vi "Create Transfer Channels.vi"(7 "direction":T1, 8 "error in (no error)":errorcluster, 9 "Transfer ID":string, 10 "Refnum in":T3, 11 "Section Ptr":T2 format="%.0x") -> (0 "error out":errorcluster)   [LabVIEW 2017, in "Data Sharing Framework System Explorer.lvlib"]
uses:
  Data Sharing Framework System Explorer.lvlib
  dsf core/Source/DSF Configuration API/1.0.0/Public/Controls/DSF Config Data RefNum.ctl
  <vilib>/NI Veristand/Custom Device API/Custom Device Item Ref.ctl
  dsf core/Source/DSF Configuration API/1.0.0/Public/Controls/DSF Direction.ctl
  <vilib>/NI Veristand/Custom Device API/Custom Device Channel Type.ctl
  <vilib>/NI Veristand/Custom Device API/Custom Device Channel.ctl
  dsf core/Source/DSF Configuration API/1.0.0/Public/Read Item Child IDs/Read Transfer Channel IDs.vi
  <vilib>/NI Veristand/Custom Device API/Custom Device API.lvlib
  dsf core/Source/DSF Configuration API/1.0.0/DSF Configuration API.lvlib
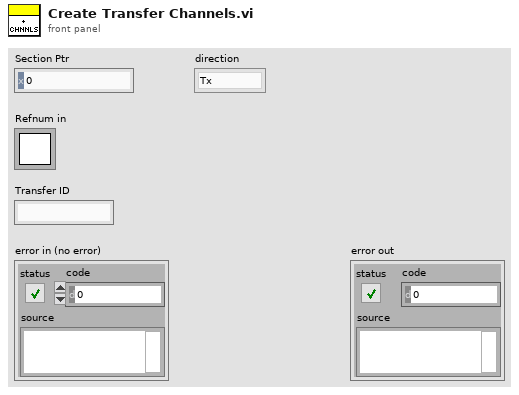
[diagram p1: front panel]
types:
  T1 = typedef "DSF Configuration API.lvlib/DSF Direction.ctl" = enum8{"Tx", "Rx"}
  T2 = typedef "Custom Device API.lvlib/Custom Device Item Ref.ctl" = u64
  T3 = typedef "DSF Configuration API.lvlib/DSF Config Data RefNum.ctl" = refnum<k1>
  T4 = typedef "Custom Device API.lvlib/Custom Device Channel Type.ctl" = enum16{"Input", "Output"}
  T5 = typedef "Custom Device API.lvlib/Custom Device Channel.ctl" = cluster{"Type":T4, "Units":string, "Default Value":dbl, "Faultable":bool, "Scalable":bool}
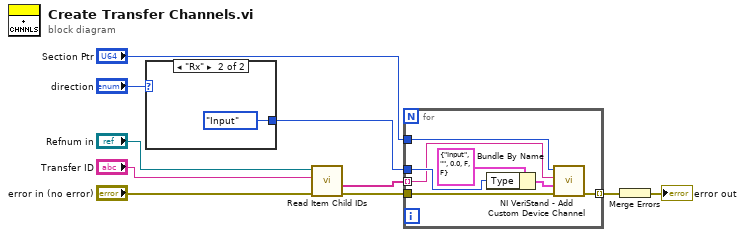
[diagram p0: block diagram]
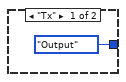
[diagram p2: hidden frame]
diagram:
  n1 = case shown="\"Rx\"" "direction" {
    tunnel: [Custom_Device_Channel_Type."Output" ("Type") Custom_Device_Channel_Type."Input" ("Type")] -> w1
    frame "Tx" {
    }
    frame "Rx" {
    }
  }
  n2 = call-poly "Read Item Child IDs.vi"("error in (no error)"="error in (no error)", "Transfer ID"="Transfer ID", "dsf refnum"="Refnum in") -> ("error out"=w4:errorcluster, "Channel IDs"=w5:string[])  [unwired: 5 in, 2 out]
  n3 = for {
    tunnel: w5 -> [w14] mode=indexing
    tunnel: w4 -> [w13]
    tunnel: [w19] -> w3 mode=indexing
    tunnel: "Section Ptr" -> [w16]
    tunnel: w1 -> [w15]
    n4 = Bundle By Name(cluster=T5 {"Type"=enum."Input", "Units"="", "Default Value"=0.0, "Faultable"=FALSE, "Scalable"=FALSE} ("Channel"), "Type"=w15) -> (w17:T5)
    n5 = call <vilib>:"NI VeriStand - Add Custom Device Channel.vi"("error in (no error)"=w13, "Channel"=w17, "Channel Name"=w14, "Parent Ref in"=w16) -> ("error out"=w19:errorcluster)  [unwired: 4 in, 3 out]
  }
  n6 = Merge Errors(w3) -> (→"error out":errorcluster)
